vi "Analysis.TestSize1DCluster.vi"() -> ()   [LabVIEW 2024]
panel:
  out "Array":T1(array[cluster])
  out "Dur(s)":dbl
  out "Cnt":i32
  out "i":i32
  in  "Count":i32
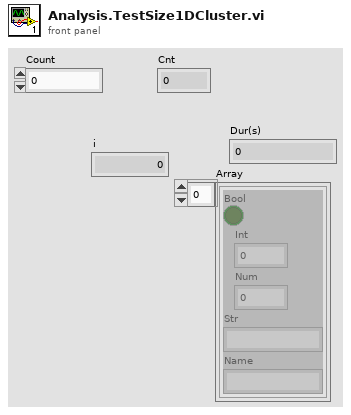
[diagram p1: front panel]
types:
  T1 = cluster{"Bool":bool, "Int":i32, "Num":dbl, "Str":string, "Name":string}[]
  T2 = cluster{"Bool":bool, "Int":i32, "Num":dbl, "Str":string, "Name":string}
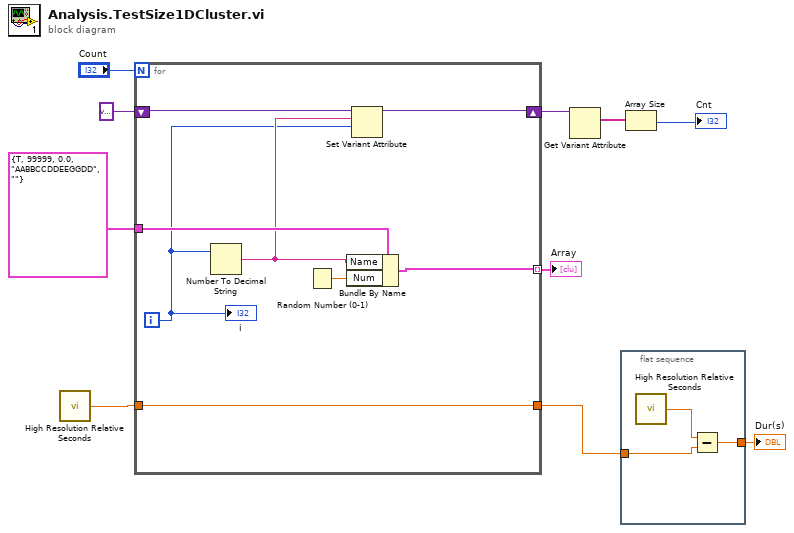
[diagram p0: block diagram]
diagram:
  n1 = call <vilib>:"High Resolution Relative Seconds.vi"() -> ("relative seconds"=w6:dbl)
  n2 = for {
    N: "Count" -> [_]
    tunnel: T2 {"Bool"=TRUE, "Int"=99999, "Num"=0.0, "Str"="AABBCCDDEEGGDD", "Name"=""} -> [w17]
    shift-right: [w14] -> w3
    shift-left: variant -> [w16]
    tunnel: w6 -> [w13]
    tunnel: [w13] -> w5
    tunnel: [w12] -> w1 mode=indexing
    i -> [w11]
    n3 = Number To Decimal String(number=w11) -> (decimal integer string=w15:string)  [unwired: 1 in]
    n4 = Random Number (0-1)() -> (number: 0 to 1=w18:dbl)
    n5 = Bundle By Name(cluster=w17, "Name"=w15, "Num"=w18) -> (w12:T2)
    n6 = Set Variant Attribute(Variant=w16, name=w15, value=w11) -> (Variant out=w14:variant)  [unwired: 1 in, 2 out]
    "i" <- w11
  }
  "Array" <- w1
  n7 = Get Variant Attribute(Variant=w3) -> (names=w4:string[])  [unwired: 3 in, 3 out]
  n8 = flat-sequence {
    tunnel: w5 -> [w20]
    tunnel: [w19] -> w7
    frame #0 {
      n9 = call <vilib>:"High Resolution Relative Seconds.vi"() -> ("relative seconds"=w21:dbl)
      n10 = Subtract(x=w21, y=w20) -> (x-y=w19:dbl)
    }
  }
  n11 = Array Size(array=w4) -> (size(s)=→"Cnt":i32)
  "Dur(s)" <- w7
